vi "XY Graph to Intensity Graph (by ref).vi"(6 "Y Label":string, 8 "error in (no error)":errorcluster, 9 "Y Scale":dbl[](array[numeric]), 11 "graph_utilities in":refnum<class "graph_utilities.lvclass">) -> (0 "error out":errorcluster, 3 "graph_utilities out":refnum<class "graph_utilities.lvclass">)   [LabVIEW 2019, in "graph_utilities.lvclass"]
doc: "Converts a sequence of XY Graphs to an Intensity Graph. Auomatically interpolates along X and Y."
uses:
  graph_utilities.lvclass
  <userlib>/LevyLab/XY Utilities/xy_utilities.lvlib
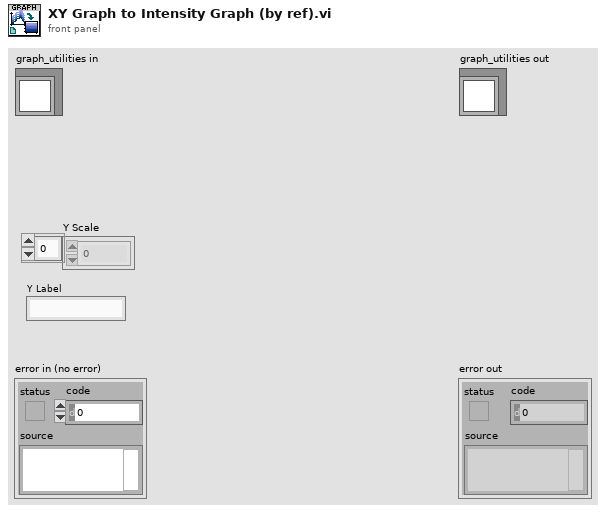
[diagram p1: front panel]
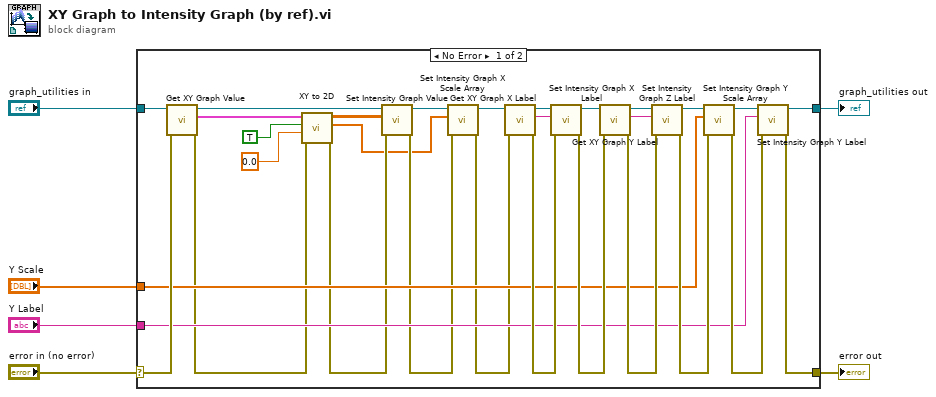
[diagram p0: block diagram]
diagram:
  n1 = case shown="No Error" "error in (no error)" {
    selector: "error in (no error)" -> [w35 w38]
    tunnel: [w21 w38] -> w5
    tunnel: [w27 w37] -> w3
    tunnel: "graph_utilities in" -> [w36 w37]
    tunnel: "Y Scale" -> [w19 _]
    tunnel: "Y Label" -> [w20 _]
    frame No Error {
      n2 = call "Get XY Graph Value.vi"("error in (no error)"=w35, "graph_utilities in"=w36) -> ("error out"=w15:errorcluster, "XY-data"=w18:cluster{"X-array":dbl[], "Y-array":dbl[]}[], "graph_utilities out"=w16:refnum<class "graph_utilities.lvclass">)  [unwired: 7 in]
      n3 = call <userlib>:"XY to 2D.vi"("error in (no error)"=w15, "Fake Point"=0.0, "Interpolate [T]"=TRUE, "XY-data"=w18) -> ("error out"=w12:errorcluster, "X Array"=w7:dbl[], "2D Y Array"=w17:dbl[][])  [unwired: 4 in, 1 out]
      n4 = call "Set Intensity Graph Value.vi"("error in (no error)"=w12, "Value"=w17, "graph_utilities in"=w16) -> ("error out"=w11:errorcluster, "graph_utilities out"=w14:refnum<class "graph_utilities.lvclass">)  [unwired: 7 in]
      n5 = call "Set Intensity Graph X Scale Array.vi"("error in (no error)"=w11, "X Scale"=w7, "graph_utilities in"=w14) -> ("error out"=w10:errorcluster, "graph_utilities out"=w13:refnum<class "graph_utilities.lvclass">)  [unwired: 7 in]
      n6 = call "Get XY Graph X Label.vi"("error in (no error)"=w10, "graph_utilities in"=w13) -> ("error out"=w26:errorcluster, "X Label"=w31:string, "graph_utilities out"=w32:refnum<class "graph_utilities.lvclass">)  [unwired: 7 in]
      n7 = call "Set Intensity Graph X Label.vi"("error in (no error)"=w26, "X Label"=w31, "graph_utilities in"=w32) -> ("error out"=w25:errorcluster, "graph_utilities out"=w30:refnum<class "graph_utilities.lvclass">)  [unwired: 7 in]
      n8 = call "Get XY Graph Y Label.vi"("error in (no error)"=w25, "graph_utilities in"=w30) -> ("error out"=w24:errorcluster, "Y Label"=w33:string, "graph_utilities out"=w34:refnum<class "graph_utilities.lvclass">)  [unwired: 7 in]
      n9 = call "Set Intensity Graph Z Label.vi"("error in (no error)"=w24, "Z Label"=w33, "graph_utilities in"=w34) -> ("error out"=w23:errorcluster, "graph_utilities out"=w29:refnum<class "graph_utilities.lvclass">)  [unwired: 7 in]
      n10 = call "Set Intensity Graph Y Scale Array.vi"("error in (no error)"=w23, "Y Scale"=w19, "graph_utilities in"=w29) -> ("error out"=w22:errorcluster, "graph_utilities out"=w28:refnum<class "graph_utilities.lvclass">)  [unwired: 7 in]
      n11 = call "Set Intensity Graph Y Label.vi"("error in (no error)"=w22, "Y Label"=w20, "graph_utilities in"=w28) -> ("error out"=w21:errorcluster, "graph_utilities out"=w27:refnum<class "graph_utilities.lvclass">)  [unwired: 7 in]
    }
    frame Error {
    }
  }
  "error out" <- w5
  "graph_utilities out" <- w3
